vi "SignalGen.vi"(6 "DSA excitation":dbl, 8 "error in (no error)":errorcluster, 9 "Enable?":bool=TRUE, 10 "Current Time [s]":dbl, 11 "Signal Cluster":T1={"phase"=0.0, "amplitude"=1.0, "frequency"=1.0, "offset"=1.0, "Signal"=enum."Sine"} {"offset" format="%0.2f"; "frequency" format="%0.2f"; "amplitude" format="%0.2f"; "phase" format="%0.2f"}) -> (0 "error out":errorcluster, 3 "Signal Out":dbl)   [LabVIEW 2017, in "SignalGen.lvlib"]
doc: "Generate Signal with various parameters"
uses:
  SignalGen.lvlib
  <vilib>/ptbypt/NI_PtbyPt.lvlib
  SignalGenParams_Cluster.ctl
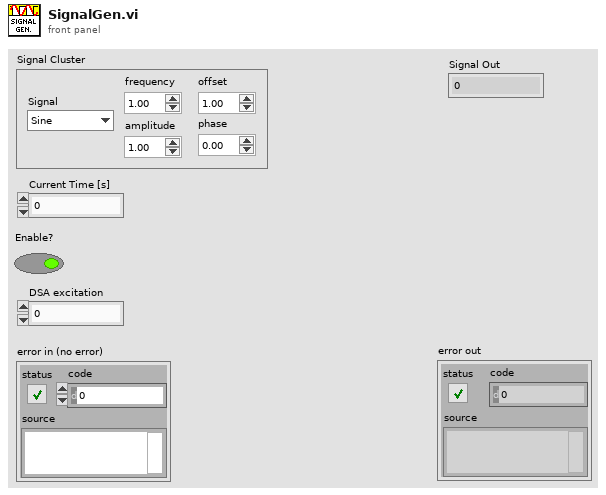
[diagram p1: front panel]
types:
  T1 = typedef "SignalGen.lvlib/SignalGenParams_Cluster.ctl" = cluster{"phase":dbl, "amplitude":dbl, "frequency":dbl, "offset":dbl, "Signal":enum16{"DC", "Sine", "Square", "Triangle", "Sawtooth", "DSA"}}
  T2 = enum16{"DC", "Sine", "Square", "Triangle", "Sawtooth", "DSA"}
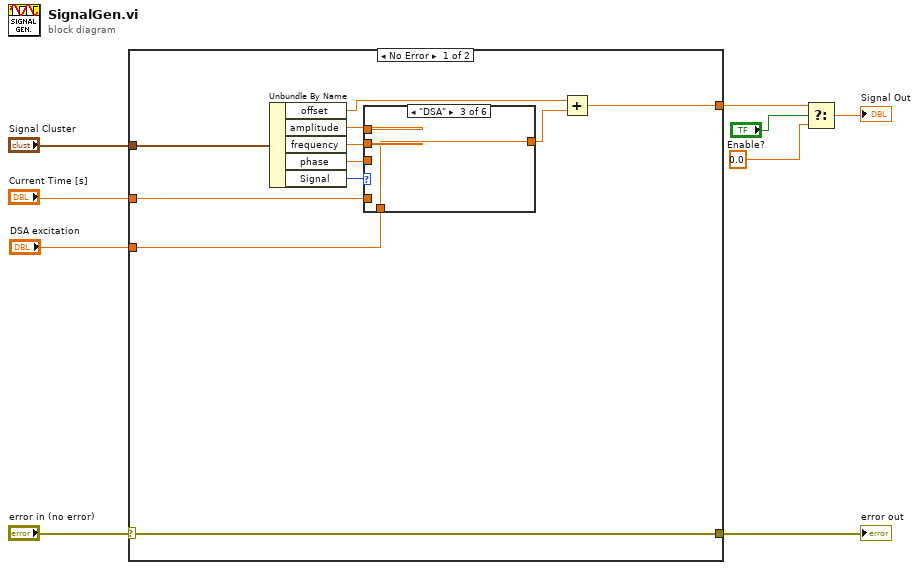
[diagram p0: block diagram]
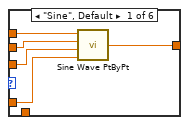
[diagram p2: hidden frame]
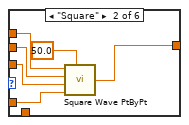
[diagram p3: hidden frame]
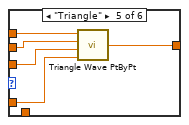
[diagram p5: hidden frame]
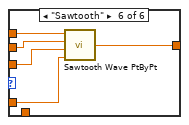
[diagram p6: hidden frame]
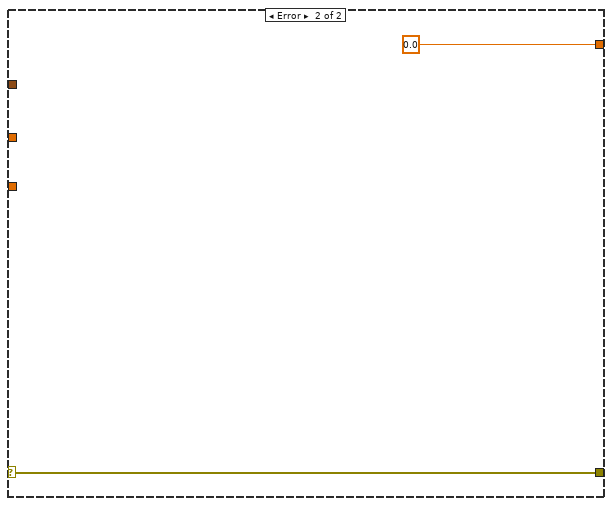
[diagram p7: hidden frame]
diagram:
  n1 = case shown="No Error" "error in (no error)" {
    selector: "error in (no error)" -> [w20 w45]
    tunnel: [w20 w45] -> w8
    tunnel: "Signal Cluster" -> [w13 _]
    tunnel: "Current Time [s]" -> [w12 _]
    tunnel: [w11 0.0] -> w5
    tunnel: "DSA excitation" -> [w10 _]
    frame No Error {
      n2 = Unbundle By Name(w13) -> ("offset"=w14:dbl, "amplitude"=w17:dbl, "frequency"=w16:dbl, "phase"=w15:dbl, "Signal"=w18:T2)
      n3 = case shown="\"DSA\"" w18 {
        tunnel: [w25 w30 w32 w33 w38 w43] -> w19
        tunnel: w17 -> [w24 w29 _ w33 w37 w42]
        tunnel: w16 -> [w23 w28 _ _ w36 w41]
        tunnel: w15 -> [w22 w27 _ _ w35 w40]
        tunnel: w12 -> [w21 w26 _ _ w34 w39]
        tunnel: w10 -> [_ _ w32 _ _ _]
        frame "Sine", Default {
          n4 = call <vilib>:"Sine Wave PtByPt.vi"("time"=w21, "phase"=w22, "frequency"=w23, "amplitude"=w24) -> ("sine wave"=w25:dbl)
        }
        frame "Square" {
          n5 = call <vilib>:"Square Wave PtByPt.vi"("amplitude"=w29, "frequency"=w28, "phase"=w27, "time"=w26, "duty cycle (%)"=50.0) -> ("square wave"=w30:dbl)
        }
        frame "DSA" {
        }
        frame "DC" {
        }
        frame "Triangle" {
          n6 = call <vilib>:"Triangle Wave PtByPt.vi"("time"=w34, "phase"=w35, "frequency"=w36, "amplitude"=w37) -> ("triangle wave"=w38:dbl)
        }
        frame "Sawtooth" {
          n7 = call <vilib>:"Sawtooth Wave PtByPt.vi"("time"=w39, "phase"=w40, "frequency"=w41, "amplitude"=w42) -> ("sawtooth wave"=w43:dbl)
        }
      }
      n8 = Add(x=w14, y=w19) -> (x+y=w11:dbl)
    }
    frame Error {
    }
  }
  "error out" <- w8
  n9 = Select(t=w5, s="Enable?", f=0.0) -> (s? t:f=→"Signal Out":dbl)
